vi "Main.vi"() -> ()   [LabVIEW 2017]
uses:
  Tag.ctl
  <vilib>/Skyline/Tag/Shared/typedefs/DataType.ctl
  <vilib>/Skyline/Tag/Wrapper/Wrapper_class/NI Skyline Tag.lvclass
  <extravilib>/ChannelInstances/Stream-c(a[.](str),a[.](bool),a[.](path))/Read With Abort.vi
  <extravilib>/ChannelInstances/Stream-c(a[.](str),a[.](bool),a[.](path))/Write With Abort.vi
  <extravilib>/ChannelInstances/Stream-c(a[.](str),a[.](bool),a[.](path))/EndpointRead.vi
  <extravilib>/ChannelInstances/Stream-c(a[.](str),a[.](bool),a[.](path))/Endpoint.vi
  <extravilib>/ChannelInstances/Stream-c(a[.](str),a[.](bool),a[.](path))/Instantiate.vi
  <extravilib>/ChannelInstances/Stream-c(a[.](str),a[.](bool),a[.](path))/)Channel.vi
  <resource>/ChannelSupport/_ChannelSupport/WaitIfNeeded.vi
  <vilib>/Skyline/Tag/Wrapper/Wrapper_class/Close Tag (Multiple).vi
  <vilib>/Skyline/Tag/Shared/NI Skyline Tag.lvlib
  <extravilib>/ChannelInstances/Stream-c(a[.](str),a[.](bool),a[.](path)).lvlib
panel:
  out "Numeric 2":i32
  out "Numeric":i32
  in  "Stop Button":bool
  in  "File Path":path=path "C:/Users/leonwei/Desktop/Data"
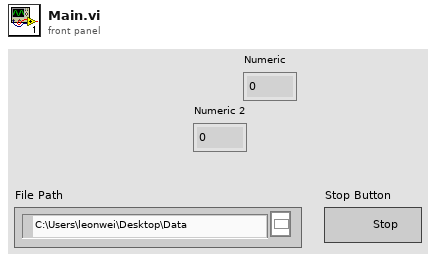
[diagram p1: front panel]
types:
  T1 = cluster{"filenames":string[], "File Change?":bool[], "File Path":path[]}
  T2 = typedef "Stream-c(a[.](str),a[.](bool),a[.](path)).lvlib/)Channel.ctl" = refnum<queue>
  T3 = typedef "Tag.ctl" = cluster{"Tag Name":string[], "Tag Type":T4[], "Tag Data":variant[], "Skyline Array":refnum<class "NI Skyline Tag.lvclass">[]}
  T4 = typedef "NI Skyline Tag.lvlib/DataType.ctl" = enum32{"Double", "I32", "String", "Boolean", "U64", "Timestamp"}
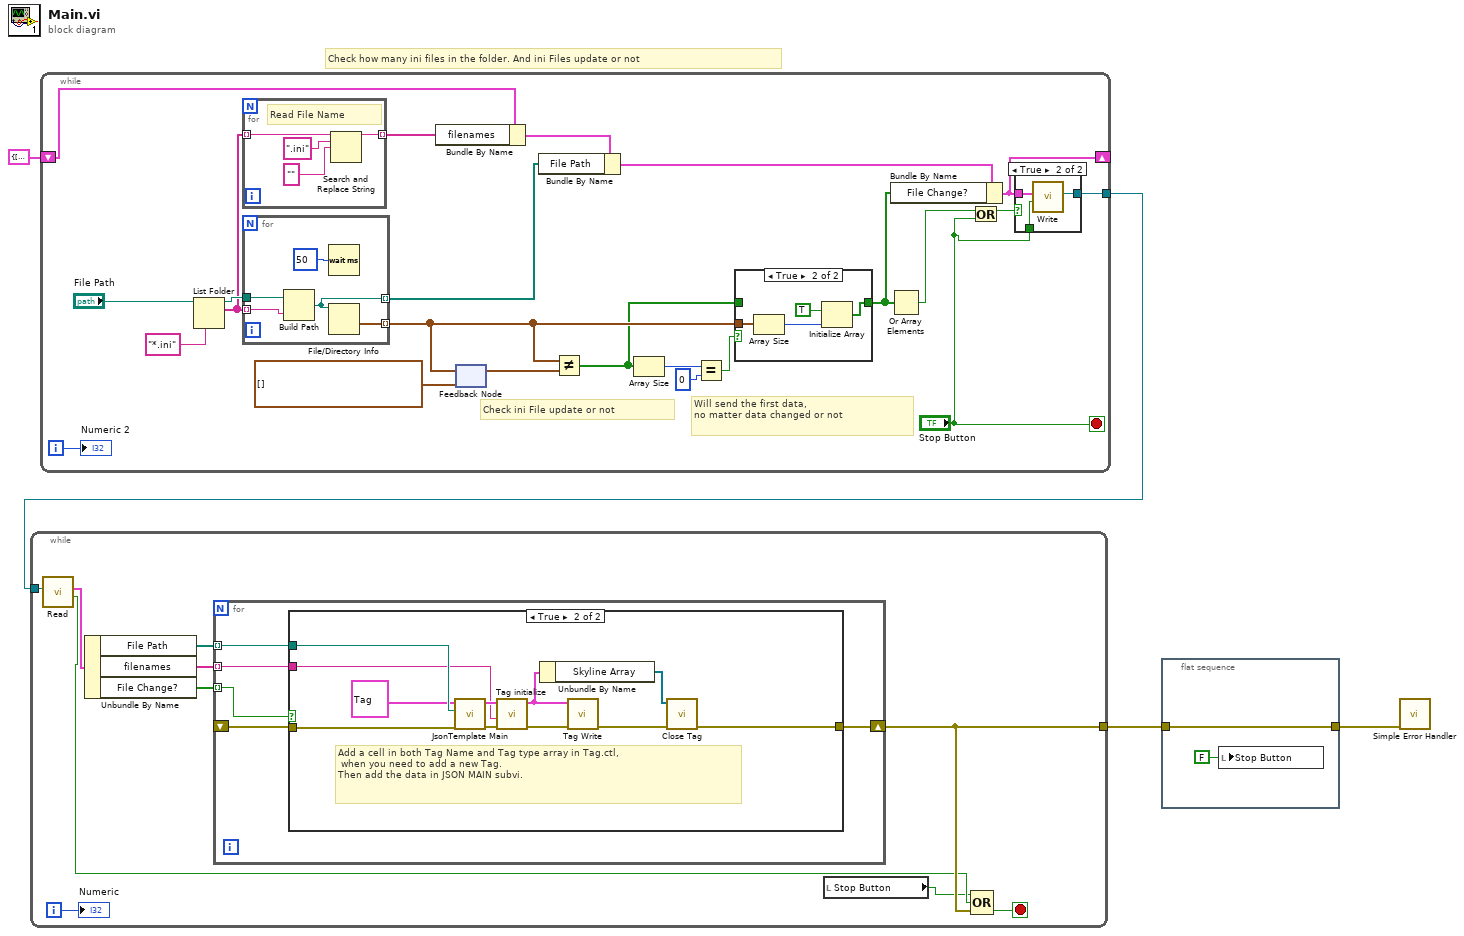
[diagram p0: block diagram]
diagram:
  # "Check how many ini files in the folder. And ini Files update or not"
  n1 = while {
    shift-right: [w21] -> _
    shift-left: T1 {"filenames"=[], "File Change?"=[FALSE, FALSE, FALSE, FALSE, FALSE], "File Path"=[]} -> [w24]
    tunnel: [w10] -> w3
    i -> [w6]
    stop <- "Stop Button" stop-if-true
    # "Will send the first data, \nno matter data changed or not"
    # "Check ini File update or not"
    n2 = List Folder(path="File Path", pattern="*.ini") -> (path out=w26:path, filenames=w25:string[])  [unwired: 2 in, 2 out]
    n3 = for {
      tunnel: w25 -> [w39] mode=indexing
      tunnel: [w36] -> w23 mode=indexing
      # "Read File Name"
      n4 = Search and Replace String(input string=w39, search string=".ini", replace string="" ("replace string (\"\")")) -> (result string=w36:string)  [unwired: 5 in, 3 out]
    }
    n5 = for {
      tunnel: w25 -> [w43] mode=indexing
      tunnel: w26 -> [w44]
      tunnel: [w42] -> w16 mode=indexing
      tunnel: [w40] -> w11 mode=indexing
      n6 = Build Path(base path=w44, name or relative path=w43) -> (appended path=w40:path)
      n7 = Wait (ms)(milliseconds to wait=u32 50) -> ()  [unwired: 1 out]
      n8 = File/Directory Info(path=w40) -> (last mod=w42:timestamp)  [unwired: 1 in, 6 out]
    }
    n9 = Bundle By Name(cluster=w24, "filenames"=w23) -> (w22:T1)
    n10 = feedback-in #1(w16) -> ()
    n11 = feedback #1(timestamp[] []) -> (w20:timestamp[])
    n12 = Bundle By Name(cluster=w22, "File Path"=w11) -> (w12:T1)
    n13 = Not Equal?(x=w16, y=w20) -> (x != y?=w15:bool[])
    n14 = Array Size(array=w15) -> (size(s)=w19:i32)
    n15 = Equal?(x=w19, y=0) -> (x = y?=w17:bool)
    n16 = case shown="True" w17 {
      tunnel: w16 -> [_ w35]
      tunnel: [w31 w32] -> w9
      tunnel: w15 -> [w31 _]
      frame False {
      }
      frame True {
        n17 = Array Size(array=w35) -> (size(s)=w34:i32)
        n18 = Initialize Array(TRUE, w34) -> (w32:bool[])
      }
    }
    n19 = Bundle By Name(cluster=w12, "File Change?"=w9) -> (w21:T1)
    n20 = Or Array Elements(Boolean array=w9) -> (logical OR=w8:bool)
    n21 = Or(x=w8, y="Stop Button") -> (x .or. y?=w7:bool)
    n22 = case shown="True" w7 {
      tunnel: w21 -> [_ w30]
      tunnel: [_ w29] -> w10
      tunnel: "Stop Button" -> [_ w28]
      frame False {
      }
      frame True {
        n23 = call <extravilib>:"Write.vi"("last element? (F)"=w28, "element"=w30) -> ("channel"=w29:T2)  [unwired: 7 in, 2 out]
      }
    }
    "Numeric 2" <- w6
  }
  n24 = while {
    tunnel: w3 -> [w51]
    tunnel: [w52] -> w2
    i -> [w48]
    stop <- w47 stop-if-true
    n25 = call <extravilib>:"Read.vi"("channel"=w51) -> ("last element?"=w46:bool, "element"=w50:T1)  [unwired: 6 in, 3 out]
    n26 = Unbundle By Name(w50) -> ("File Path"=w49:path[], "filenames"=w54:string[], "File Change?"=w53:bool[])
    n27 = for {
      tunnel: w54 -> [w57] mode=indexing
      tunnel: w53 -> [w58] mode=indexing
      shift-right: [w59] -> w52
      shift-left: _ -> [w55]
      tunnel: w49 -> [w56] mode=indexing
      n28 = case shown="True" w58 {
        tunnel: [w60 w66] -> w59
        tunnel: w57 -> [_ w64]
        tunnel: w56 -> [_ w65]
        tunnel: w55 -> [w60 w63]
        frame False {
        }
        frame True {
          # "Add a cell in both Tag Name and Tag type array in Tag.ctl,\n when you need to add a new Tag. \nThen add the data in JSON MAIN subvi."
          n29 = call "JsonTemplate Main.vi"("Error In"=w63, "file (use dialog)"=w65, "Tag IN"=T3 {"Tag Name"=["LStatus", "RStatus", "LTargetTemp", "LTemp1", "LTemp2", "LTemp3", "LTemp4", "LTemp5", "LTemp6", "RTargetT", "RTemp1", "RTemp2", "RTemp3", "RTemp4", "RTemp5", "RTemp6", "LWO", "LOPID", "LDate", "LTime", "LModel", "LAgingTime", "LAgingTemp", "LStartTime", "LEndTime", "RWO", "ROPID", "RDate", "RTime", "RModel", "RAgingTime", "RAgingTemp", "RStartTime", "REndTime", "TempWarning"], "Tag Type"=[enum."String", enum."String", enum."Double", enum."Double", enum."Double", enum."Double", enum."Double", enum."Double", enum."Double", enum."Double", enum."Double", enum."Double", enum."Double", enum."Double", enum."Double", enum."Double", enum."String", enum."String", enum."String", enum."String", enum."String", enum."String", enum."String", enum."String", enum."String", enum."String", enum."String", enum."String", enum."String", enum."String", enum."String", enum."String", enum."String", enum."String", enum."Boolean"], "Tag Data"=[], "Skyline Array"=[]} ("Cluster")) -> ("Error Out"=w62:errorcluster, "TAG  Out"=w71:T3)  [unwired: 7 in]
          n30 = call "Tag initialize.vi"("error In"=w62, "namespace"=w64, "Tag IN"=w71) -> ("error out"=w68:errorcluster, "output cluster"=w70:T3)  [unwired: 7 in]
          n31 = Unbundle By Name(w70) -> ("Skyline Array"=w69:refnum<class "NI Skyline Tag.lvclass">[])
          n32 = call "Tag Write.vi"("error in (no error)"=w68, "Tag IN"=w70) -> ("error out"=w67:errorcluster)  [unwired: 9 in]
          n33 = call-poly <vilib>:"Close Tag.vi"("error in (no error)"=w67, "tags in"=w69) -> ("error out"=w66:errorcluster)  [unwired: 9 in]
        }
      }
    }
    n34 = local read "Stop Button"() -> (w45:bool)
    n35 = Compound Arithmetic op=OR(w45, w46, w52) -> (w47:bool)
    "Numeric" <- w48
  }
  n36 = flat-sequence {
    tunnel: w2 -> [w73]
    tunnel: [w73] -> w1
    frame #0 {
      n37 = local write "Stop Button"(FALSE ("Stop Button")) -> ()
    }
  }
  n38 = call <vilib>:"Simple Error Handler.vi"("error in (no error)"=w1) -> ()  [unwired: 4 in, 5 out]
